vi "fg_vi_reference.vi"(7 "command":T1=enum."read", 8 "error in (no error)":errorcluster, 11 "vi_reference in":refnum<vi>) -> (0 "error out":errorcluster, 3 "vi_reference out":refnum<vi>)   [LabVIEW 2015, in "lv-recipe-machine.lvlib"]
uses:
  lv-recipe-machine.lvlib
  _controls/fg_command.ctl
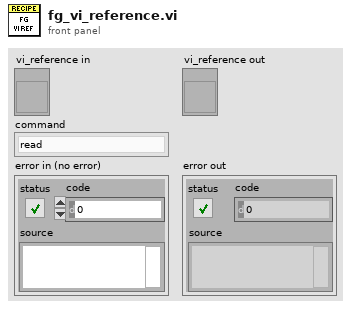
[diagram p1: front panel]
types:
  T1 = typedef "lv-recipe-machine.lvlib/fg_command.ctl" = enum16{"<fg_command>", "initialize", "read", "write", "shutdown", "<null>"}
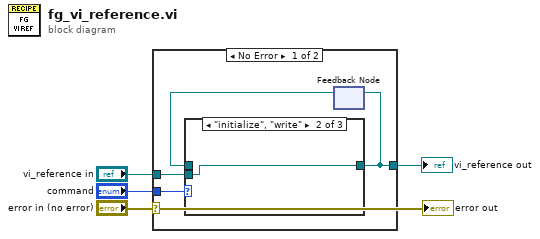
[diagram p0: block diagram]
diagram:
  n1 = case shown="No Error" "error in (no error)" {
    tunnel: "command" -> [w8 _]
    tunnel: "vi_reference in" -> [w7 _]
    tunnel: [w5 _] -> w1
    frame No Error {
      n2 = feedback #1() -> (w6:refnum<vi>)  [unwired: 1 in]
      n3 = case shown="\"initialize\", \"write\"" w8 {
        tunnel: w7 -> [_ w10 _]
        tunnel: [w9 w10 _] -> w5
        tunnel: w6 -> [w9 _ _]
        frame Default {
        }
        frame "initialize", "write" {
        }
        frame "shutdown" {
        }
      }
      n4 = feedback-in #1(w5) -> ()
    }
    frame Error {
    }
  }
  "vi_reference out" <- w1
  "error out" <- "error in (no error)"
